vi "Control - Set Settings.vi"(8 "error in (no error)":errorcluster, 11 "Folder Path":path) -> (0 "error out":errorcluster)   [LabVIEW 2017]
uses:
  <vilib>/Utility/miscctls.llb/LVPositionTypeDef.ctl
  <vilib>/Utility/miscctls.llb/LVRectTypeDef.ctl
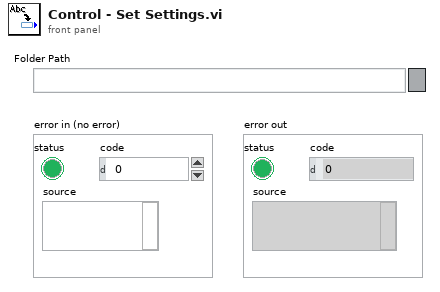
[diagram p1: front panel]
types:
  T1 = typedef "LVRectTypeDef.ctl" = cluster{"Left":i16, "Top":i16, "Right":i16, "Bottom":i16}
  T2 = typedef "LVPositionTypeDef.ctl" = cluster{"Left":i32, "Top":i32}
  T3 = typedef "imagedata.ctl" = cluster{"image type":i32, "image depth":i32, "image":u8[], "mask":u8[], "colors":u32[], "Rectangle":cluster{"left":i16, "top":i16, "right":i16, "bottom":i16}}
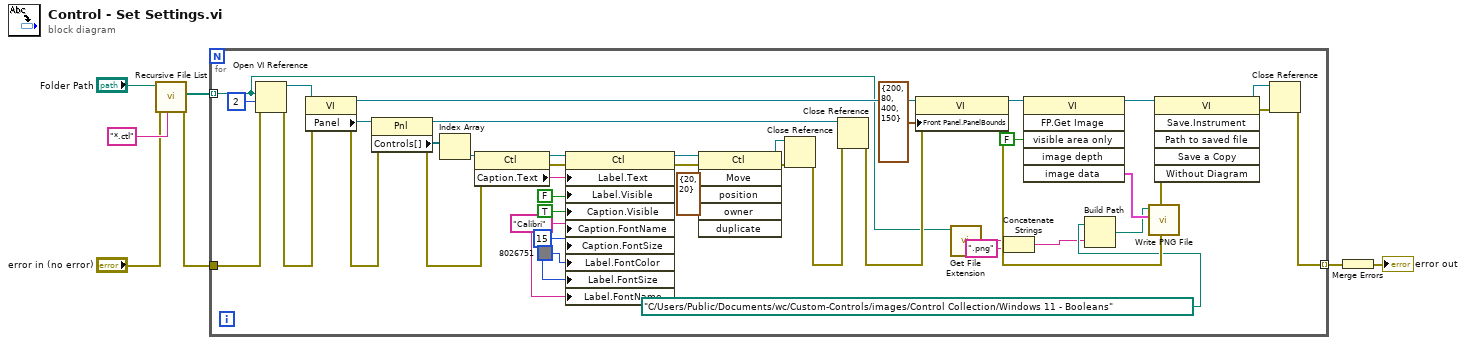
[diagram p0: block diagram]
diagram:
  n1 = call <vilib>:"Recursive File List.vi"("pattern"="*.ctl", "error in (no error)"="error in (no error)", "Folder Path"="Folder Path") -> ("error out"=w3:errorcluster, "All Files in Dir"=w4:path[])  [unwired: 4 in, 3 out]
  n2 = for {
    tunnel: w4 -> [w12] mode=indexing
    tunnel: w3 -> [w39]
    tunnel: [w34] -> w2 mode=indexing
    w33 = "Calibri" ("Font Name")
    w31 = u16 15 ("Size")
    n3 = Open VI Reference(vi path=w12, options=2, error in (no error)=w39) -> (vi reference=w47:refnum<vi>, error out=w46:errorcluster)  [unwired: 3 in]
    n4 = property class="VI"(reference=w47, error in=w46) -> (reference out=w17:refnum<vi>, error out=w40:errorcluster, "Panel"=w45:refnum<vi>)
    n5 = property class="Pnl"(reference=w45, error in=w40) -> (reference out=w38:refnum<vi>, error out=w28:errorcluster, "Controls[]"=w44:refnum<vi>[])
    n6 = Index Array(array=w44) -> (element=w43:refnum<vi>)  [unwired: 1 in]
    n7 = property class="Ctl"(reference=w43, error in=w28) -> (reference out=w30:refnum<vi>, error out=w27:errorcluster, "Caption.Text"=w29:string)
    n8 = property class="Ctl"(reference=w30, error in=w27, "Label.Text"=w29, "Label.Visible"=FALSE, "Caption.Visible"=TRUE, "Caption.FontName"=w33, "Caption.FontSize"=w31, "Label.FontColor"=u32 8026751 ("Color"), "Label.FontSize"=w31, "Label.FontName"=w33) -> (reference out=w26:refnum<vi>, error out=w24:errorcluster)
    n9 = invoke class="Ctl" method="Move"(reference=w26, error in=w24, "position"=T2 {"Left"=20, "Top"=20}) -> (reference out=w25:refnum<vi>, error out=w23:errorcluster)  [unwired: 3 in, 4 out]
    n10 = Close Reference(reference=w25, error in (no error)=w23) -> (error out=w37:errorcluster)
    n11 = Close Reference(reference=w38, error in (no error)=w37) -> (error out=w20:errorcluster)
    n12 = property class="VI"(reference=w17, error in=w20, "Front Panel.PanelBounds"=T1 {"Left"=200, "Top"=80, "Right"=400, "Bottom"=150} ("Front Panel Window:Panel Bounds")) -> (reference out=w16:refnum<vi>, error out=w19:errorcluster)
    n13 = call <vilib>:"Get File Extension.vi"("file"=w12) -> ("filename without extension"=w11:string)  [unwired: 6 in, 4 out]
    n14 = Concatenate Strings(w11, ".png" ("string")) -> (w10:string)
    n15 = invoke class="VI" method="FP.Get Image"(reference=w16, "visible area only"=FALSE ("Visible Area Only")) -> (reference out=w15:refnum<vi>, "image data"=w18:T3)  [unwired: 4 in, 4 out]
    n16 = Build Path(base path=path "C:/Users/Public/Documents/wc/Custom-Controls/images/Control Collection/Windows 11 - Booleans", name or relative path=w10) -> (appended path=w13:path)
    n17 = call <vilib>:"Write PNG File.vi"("image data"=w18, "path to PNG file"=w13) -> ()  [unwired: 8 in, 2 out]
    n18 = invoke class="VI" method="Save.Instrument"(reference=w15, error in=w19) -> (reference out=w36:refnum<vi>, error out=w35:errorcluster)  [unwired: 4 in, 4 out]
    n19 = Close Reference(reference=w36, error in (no error)=w35) -> (error out=w34:errorcluster)
  }
  n20 = Merge Errors(w2) -> (→"error out":errorcluster)
